vi "test.vi"   [LabVIEW 2019]
uses:
  <vilib>/Utility/config.llb/NI_LVConfig.lvlib
  <vilib>/Utility/config.llb/Write Key (Boolean).vi
types:
  T1 = typedef "NI_LVConfig.lvlib/Config Data RefNum.ctl" = refnum<k1>
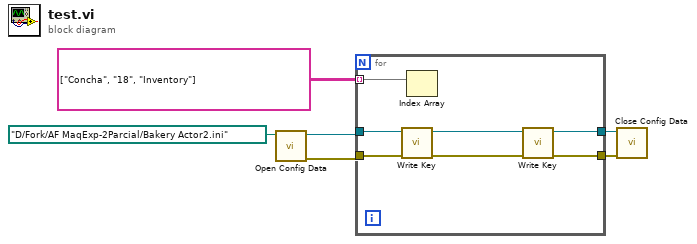
[diagram p0: block diagram]
diagram:
  n1 = call <vilib>:"Open Config Data.vi"("configuration file path"=path "D:/Fork/AF MaqExp-2Parcial/Bakery Actor2.ini") -> ("error out"=w3:errorcluster, "refnum"=w4:T1)  [unwired: 8 in, 1 out]
  n2 = for {
    tunnel: w4 -> [w9]
    tunnel: [w10] -> w5
    tunnel: w3 -> [w8]
    tunnel: [w11] -> w6
    tunnel: string[][] [["Concha", "18", "Inventory"]] -> [w7] mode=indexing
    n3 = call-poly <vilib>:"Write Key.vi"("error in (no error)"=w8, "refnum"=w9) -> ("error out"=w13:errorcluster, "refnum out"=w12:T1)  [unwired: 7 in, 1 out]
    n4 = Index Array(array=w7) -> ()  [unwired: 1 in, 1 out]
    n5 = call-poly <vilib>:"Write Key.vi"("error in (no error)"=w13, "refnum"=w12) -> ("error out"=w11:errorcluster, "refnum out"=w10:T1)  [unwired: 7 in, 1 out]
  }
  n6 = call <vilib>:"Close Config Data.vi"("error in (no error)"=w6, "refnum"=w5) -> ()  [unwired: 8 in, 2 out]
